vi "FlipBit(U8).vi"(8 "error in (no error)":errorcluster caption="错误输入（无错误）", 10 "Bit(0-7)":u8, 11 "Input(U8)":u8 format="%.0x") -> (0 "error out":errorcluster caption="错误输出", 3 "Output(U8)":u8 format="%.0x")   [LabVIEW 2011]
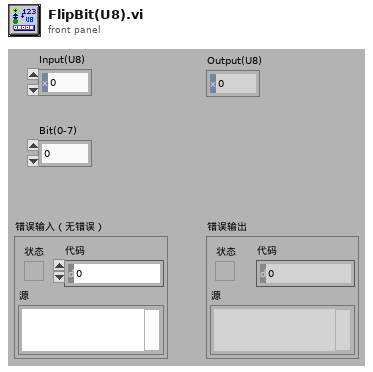
[diagram p1: front panel]
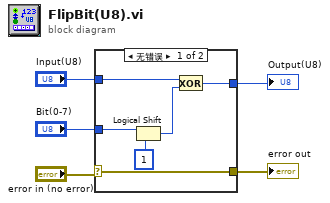
[diagram p0: block diagram]
diagram:
  n1 = case shown="无错误" "error in (no error)" {
    selector: "error in (no error)" -> [w11 w12]
    tunnel: [w11 w12] -> w4
    tunnel: "Bit(0-7)" -> [w9 _]
    tunnel: "Input(U8)" -> [w8 _]
    tunnel: [w6 _] -> w1
    frame No Error {
      n2 = Logical Shift(y=w9, x=u8 1) -> (x << y=w7:u8)
      n3 = Exclusive Or(1:w7, 2:w8) -> (0:w6:u8)
    }
    frame Error {
    }
  }
  "error out" <- w4
  "Output(U8)" <- w1
